vi "100kHz PID - PipelinedIsolation.vi"() -> ()   [LabVIEW 2010]
uses:
  <vilib>/eio/EIONode/EIONode.xnode
  <vilib>/rvi/eio/nirviEIOImplementation/nirviEIOImplementation.xnode
  <vilib>/rvi/eio/common/nirviEmuClasses.ctl
  <vilib>/addons/control/pid/fpga.llb/XNode/niFpgaPID.xnode
  <vilib>/rvi/eio/common/nirviEmuTemplateMethod_noerrors.vi
panel:
  in  "PID.Setpoint.PID 2":i16
  in  "PID.Proportional Gain.PID 2":i16=1
  in  "PID.Integral Gain.PID 2":i16
  in  "PID.Derivative Gain.PID 2":i16
  in  "PID.Setpoint.PID 3":i16
  in  "PID.Proportional Gain.PID 3":i16=1
  in  "PID.Integral Gain.PID 3":i16
  in  "PID.Derivative Gain.PID 3":i16
  out "PID.Num Ticks":u32
  in  "PID.Setpoint.PID 1":i16
  in  "PID.Proportional Gain.PID 1":i16=1
  in  "PID.Integral Gain.PID 1":i16
  in  "PID.Derivative Gain.PID 1":i16
  in  "PID.Setpoint.PID 0":i16
  in  "PID.Proportional Gain.PID 0":i16=1
  in  "PID.Integral Gain.PID 0":i16
  in  "PID.Derivative Gain.PID 0":i16
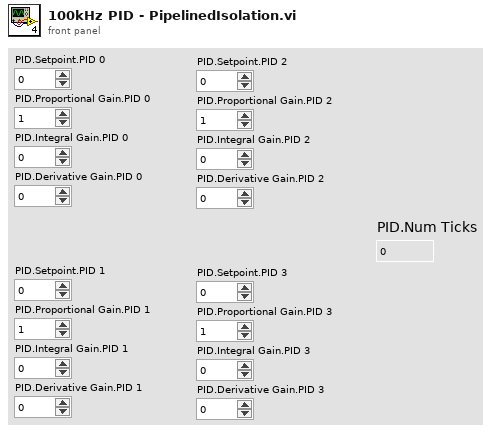
[diagram p1: front panel]
types:
  T1 = cluster{"proportional gain (Kc)":i16, "integral gain (Kc*Ts/Ti)":i16, "derivative gain (Kc*Td/Ts)":i16}
  T2 = typedef "nirviEmuClasses.ctl" = enum16{"IO Read", "IO Write", "Method", "Property Read", "Property Write"}
  T3 = cluster{"proportional gain (Kc)":fxp<+/-,16,8>, "proportional gain (Kc)":fxp<+/-,16,8>, "proportional gain (Kc)":fxp<+/-,16,8>}
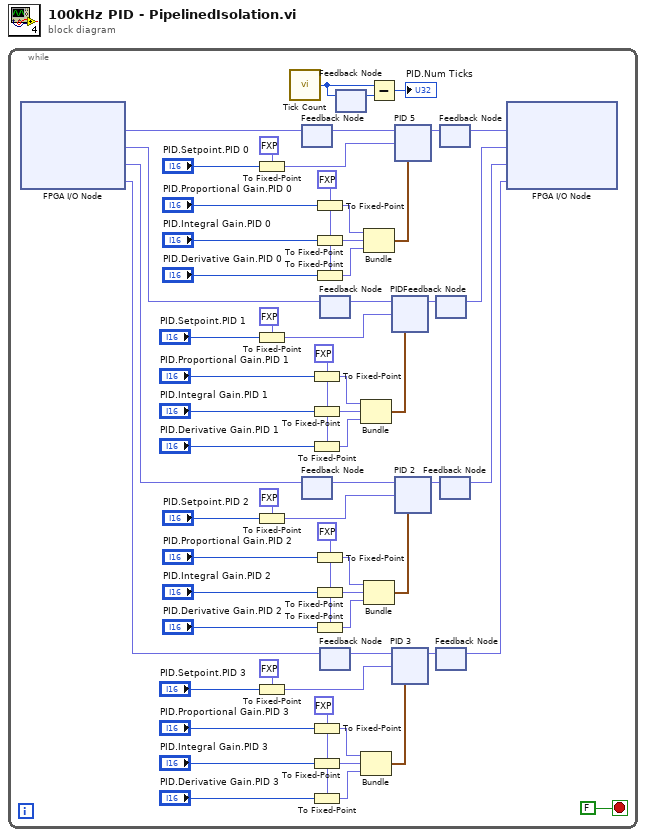
[diagram p0: block diagram]
diagram:
  n1 = while {
    stop <- FALSE stop-if-true
    w23 = fxp<+/-,16,8> 0.0 ("proportional gain (Kc)")
    w12 = fxp<+/-,16,8> 0.0 ("proportional gain (Kc)")
    w40 = fxp<+/-,16,8> 0.0 ("proportional gain (Kc)")
    w57 = fxp<+/-,16,8> 0.0 ("proportional gain (Kc)")
    n2 = xnode "FPGA I/O Node"() -> ("NI 9215/AI0"=w50:fxp<+/-,20,5>, "NI 9215/AI1"=w31:fxp<+/-,20,5>, "NI 9215/AI2"=w3:fxp<+/-,20,5>, "NI 9215/AI3"=w4:fxp<+/-,20,5>)  [unwired: 4 in, 4 out]
    n3 = To Fixed-Point(fixed-point type=fxp<+/-,16,5> 0.0 ("setpoint"), number="PID.Setpoint.PID 0") -> (fixed-point=w53:fxp<+/-,16,5>)
    n4 = To Fixed-Point(fixed-point type=fxp<+/-,16,5> 0.0 ("setpoint"), number="PID.Setpoint.PID 1") -> (fixed-point=w42:fxp<+/-,16,5>)
    n5 = To Fixed-Point(fixed-point type=fxp<+/-,16,5> 0.0 ("setpoint"), number="PID.Setpoint.PID 2") -> (fixed-point=w15:fxp<+/-,16,5>)
    n6 = To Fixed-Point(fixed-point type=fxp<+/-,16,5> 0.0 ("setpoint"), number="PID.Setpoint.PID 3") -> (fixed-point=w21:fxp<+/-,16,5>)
    n7 = call "Tick Count"() -> ("Tick Count(Ticks)"=w48:u32)
    n8 = feedback-in #1(w50) -> ()
    n9 = feedback #1() -> (w46:fxp<+/-,20,5>)  [unwired: 1 in]
    n10 = feedback #2() -> (w17:fxp<+/-,20,5>)  [unwired: 1 in]
    n11 = feedback-in #2(w3) -> ()
    n12 = To Fixed-Point(fixed-point type=w40, number="PID.Proportional Gain.PID 1") -> (fixed-point=w37:fxp<+/-,16,8>)
    n13 = To Fixed-Point(fixed-point type=w40, number="PID.Integral Gain.PID 1") -> (fixed-point=w38:fxp<+/-,16,8>)
    n14 = To Fixed-Point(fixed-point type=w40, number="PID.Derivative Gain.PID 1") -> (fixed-point=w39:fxp<+/-,16,8>)
    n15 = To Fixed-Point(fixed-point type=w23, number="PID.Proportional Gain.PID 3") -> (fixed-point=w26:fxp<+/-,16,8>)
    n16 = To Fixed-Point(fixed-point type=w23, number="PID.Integral Gain.PID 3") -> (fixed-point=w25:fxp<+/-,16,8>)
    n17 = To Fixed-Point(fixed-point type=w23, number="PID.Derivative Gain.PID 3") -> (fixed-point=w24:fxp<+/-,16,8>)
    n18 = To Fixed-Point(fixed-point type=w57, number="PID.Proportional Gain.PID 0") -> (fixed-point=w60:fxp<+/-,16,8>)
    n19 = To Fixed-Point(fixed-point type=w57, number="PID.Integral Gain.PID 0") -> (fixed-point=w59:fxp<+/-,16,8>)
    n20 = To Fixed-Point(fixed-point type=w57, number="PID.Derivative Gain.PID 0") -> (fixed-point=w58:fxp<+/-,16,8>)
    n21 = To Fixed-Point(fixed-point type=w12, number="PID.Proportional Gain.PID 2") -> (fixed-point=w9:fxp<+/-,16,8>)
    n22 = To Fixed-Point(fixed-point type=w12, number="PID.Integral Gain.PID 2") -> (fixed-point=w10:fxp<+/-,16,8>)
    n23 = To Fixed-Point(fixed-point type=w12, number="PID.Derivative Gain.PID 2") -> (fixed-point=w11:fxp<+/-,16,8>)
    n24 = feedback #3() -> (w45:fxp<+/-,20,5>)  [unwired: 1 in]
    n25 = feedback-in #3(w31) -> ()
    n26 = feedback #4() -> (w18:fxp<+/-,20,5>)  [unwired: 1 in]
    n27 = feedback-in #4(w4) -> ()
    n28 = feedback-in #5(w48) -> ()
    n29 = feedback #5() -> (w49:u32)  [unwired: 1 in]
    n30 = Bundle("proportional gain (Kc)"=w37, "proportional gain (Kc)"=w38, "proportional gain (Kc)"=w39) -> (w36:T3)  [unwired: 1 in]
    n31 = Bundle("proportional gain (Kc)"=w26, "proportional gain (Kc)"=w25, "proportional gain (Kc)"=w24) -> (w27:T3)  [unwired: 1 in]
    n32 = Bundle("proportional gain (Kc)"=w60, "proportional gain (Kc)"=w59, "proportional gain (Kc)"=w58) -> (w61:T3)  [unwired: 1 in]
    n33 = Bundle("proportional gain (Kc)"=w9, "proportional gain (Kc)"=w10, "proportional gain (Kc)"=w11) -> (w8:T3)  [unwired: 1 in]
    n34 = Subtract(x=w48, y=w49) -> (x-y=→"PID.Num Ticks":u32)
    n35 = xnode ("PID")("process variable"=w45, "setpoint"=w42, "PID gains"=w36) -> ("output"=w44:fxp<+/-,16,5>)  [unwired: 2 in]
    n36 = xnode ("PID 3")("process variable"=w18, "setpoint"=w21, "PID gains"=w27) -> ("output"=w19:fxp<+/-,16,5>)  [unwired: 2 in]
    n37 = xnode ("PID 5")("process variable"=w46, "setpoint"=w53, "PID gains"=w61) -> ("output"=w52:fxp<+/-,16,5>)  [unwired: 2 in]
    n38 = xnode ("PID 2")("process variable"=w17, "setpoint"=w15, "PID gains"=w8) -> ("output"=w16:fxp<+/-,16,5>)  [unwired: 2 in]
    n39 = feedback #6() -> (w32:fxp<+/-,16,5>)  [unwired: 1 in]
    n40 = feedback-in #6(w44) -> ()
    n41 = feedback #7() -> (w2:fxp<+/-,16,5>)  [unwired: 1 in]
    n42 = feedback-in #7(w19) -> ()
    n43 = feedback-in #8(w52) -> ()
    n44 = feedback #8() -> (w51:fxp<+/-,16,5>)  [unwired: 1 in]
    n45 = feedback #9() -> (w1:fxp<+/-,16,5>)  [unwired: 1 in]
    n46 = feedback-in #9(w16) -> ()
    n47 = xnode "FPGA I/O Node"("NI 9269/AO0"=w51, "NI 9269/AO1"=w32, "NI 9269/AO2"=w1, "NI 9269/AO3"=w2) -> ()  [unwired: 4 in, 4 out]
  }
